vi "deadband.vi"(1 "joystick axis":dbl(slide)=nan min=-1.0 max=1.0 step=0.01 scale=-1.0..1.0, 2 "Deadband":dbl) -> (0 "deadbanded_output":dbl)   [LabVIEW 2017]
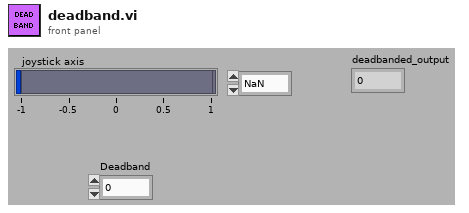
[diagram p1: front panel]
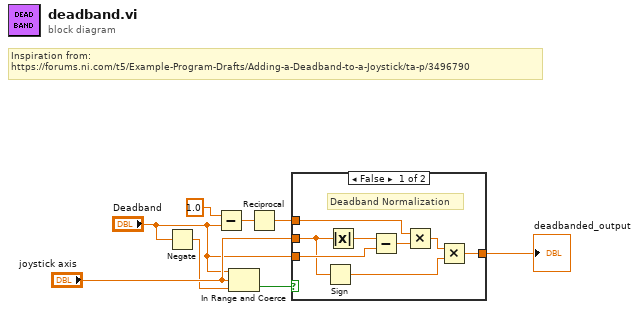
[diagram p0: block diagram]
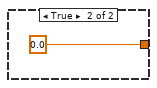
[diagram p2: hidden frame]
diagram:
  # "Inspiration from:\nhttps://forums.ni.com/t5/Example-Program-Drafts/Adding-a-Deadband-to-a-Joystick/ta-p/3496790"
  n1 = Negate(x="Deadband") -> (-x=w6:dbl)
  n2 = Subtract(x=1.0, y="Deadband") -> (x-y=w3:dbl)
  n3 = In Range and Coerce(upper limit="Deadband", x="joystick axis", lower limit=w6) -> (In Range?=w5:bool)  [unwired: 1 out]
  n4 = Reciprocal(x=w3) -> (1/x=w2:dbl)
  n5 = case shown="False" w5 {
    tunnel: "joystick axis" -> [w11 _]
    tunnel: [w10 0.0 ("Left Side")] -> w7
    tunnel: "Deadband" -> [w12 _]
    tunnel: w2 -> [w9 _]
    frame False {
      # "Deadband Normalization"
      n6 = Sign(1:w11) -> (0:w14:dbl)
      n7 = Absolute Value(x=w11) -> (abs(x)=w16:dbl)
      n8 = Subtract(x=w16, y=w12) -> (x-y=w15:dbl)
      n9 = Multiply(x=w9, y=w15) -> (x*y=w13:dbl)
      n10 = Multiply(x=w13, y=w14) -> (x*y=w10:dbl)
    }
    frame True {
    }
  }
  "deadbanded_output" <- w7
